vi "Update square wave frequency.vi"(8 "Error In":errorcluster, 10 "Frequency":dbl=100.0 min=100.0 max=10000.0 step=1.0 format="%#_g Hz", 11 "Arduino Port":refnum<visa-resource-name>) -> (0 "Error Out":errorcluster, 3 "Arduino Port out":refnum<visa-resource-name>)   [LabVIEW 2016]
doc: "Perform an update of the voltage output of the input channel of AD5535. The max speed of this operation is 1-2ms"
uses:
  Typedef/AD5535 - Command.ctl
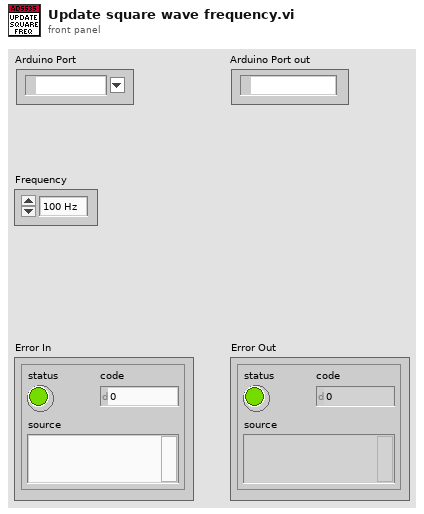
[diagram p1: front panel]
types:
  T1 = typedef "AD5535 - Command.ctl" = enum16{"None", "Start", "Stop", "Load Array", "Update channel", "Update frequency", "Prova"}
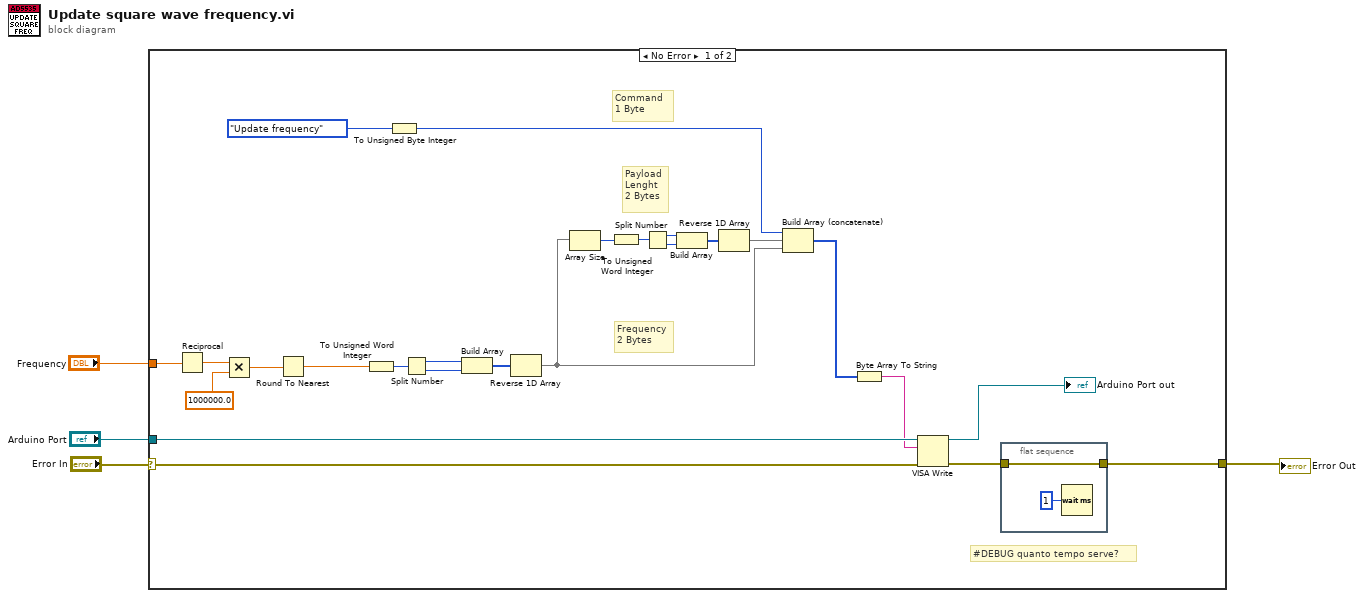
[diagram p0: block diagram]
diagram:
  n1 = case shown="No Error" "Error In" {
    selector: "Error In" -> [w28 w32]
    tunnel: [w25 w32] -> w3
    tunnel: "Arduino Port" -> [w29 _]
    tunnel: "Frequency" -> [w6 _]
    frame No Error {
      # "Frequency\n2 Bytes"
      # "Command\n1 Byte"
      # "Payload\nLenght\n2 Bytes"
      # "#DEBUG quanto tempo serve?"
      n2 = Reciprocal(x=w6) -> (1/x=w7:dbl)
      n3 = Multiply(x=w7, y=1000000.0) -> (x*y=w9:dbl)
      n4 = Round To Nearest(number=w9) -> (nearest integer value=w10:dbl)
      n5 = To Unsigned Word Integer(number=w10) -> (unsigned 16bit integer=w11:u16)
      n6 = To Unsigned Byte Integer(number=AD5535_-_Command."Update frequency" ("AD5535 - Command")) -> (unsigned 8bit integer=w23:u8)
      n7 = Split Number(x=w11) -> (hi(x)=w12:u8, lo(x)=w13:u8)
      n8 = Build Array(w12, w13) -> (w14:u8[])
      n9 = Reverse 1D Array(array=w14) -> (reversed array=w5:u8[])
      n10 = Array Size(array=w5) -> (size(s)=w18:i32)
      n11 = To Unsigned Word Integer(number=w18) -> (unsigned 16bit integer=w19:u16)
      n12 = Split Number(x=w19) -> (hi(x)=w20:u8, lo(x)=w21:u8)
      n13 = Build Array(w20, w21) -> (w22:u8[])
      n14 = Reverse 1D Array(array=w22) -> (reversed array=w17:u8[])
      n15 = Build Array (concatenate)(w23, w17, w5) -> (w16:u8[])
      n16 = Byte Array To String(unsigned byte array=w16) -> (string=w15:string)
      n17 = VISA Write(VISA resource name=w29, write buffer=w15, error in (no error)=w28) -> (VISA resource name out=→"Arduino Port out":refnum<visa-resource-name>, error out=w26:errorcluster)  [unwired: 1 out]
      n18 = flat-sequence {
        tunnel: w26 -> [w31]
        tunnel: [w31] -> w25
        frame #0 {
          n19 = Wait (ms)(milliseconds to wait=u32 1) -> ()  [unwired: 1 out]
        }
      }
    }
    frame Error {
    }
  }
  "Error Out" <- w3
